vi "Open Server.vi"   [LabVIEW 2020, in "NI_DataFinder.lvlib"]
doc: "Connects a DataFinder or a DataFinder federation with the specified connection parameters."
uses:
  <vilib>/DataFinder/NI_DataFinder.lvlib
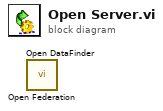
[diagram p0: block diagram]
diagram:
  n1 = call <vilib>:"Open Federation.vi"() -> ()  [unwired: 14 in, 2 out]
  n2 = call <vilib>:"Open DataFinder.vi"() -> ()  [unwired: 14 in, 2 out]
